vi "Begin.vi"(8 "error in":errorcluster) -> (0 "error out":errorcluster)   [LabVIEW 2018]
doc: "Called before other user functions, this VI is expected to open initial I/O refnums, load in file data, and do all program initialization. Notice that the <B>error out</B> terminal is simply used for data flow. Wiring it to other structures or subVIs ensures that this VI runs first."
uses:
  <vilib>/Rock Robotics/WPI/DriverStation/WPI_DriverStationRobotMode2.ctl
  <vilib>/Rock Robotics/WPI/Joystick/WPI_JoystickDeviceEnum.ctl
  <vilib>/Rock Robotics/WPI/Solenoid/WPI_SolenoidChannel.ctl
  <vilib>/Rock Robotics/SystemInterfaces/DIO/FPGA_DIOPWMChannel.ctl
  <vilib>/Rock Robotics/SystemInterfaces/AI/FPGA_AIChannel.ctl
  <vilib>/Rock Robotics/SystemInterfaces/spilib/spi_bus.ctl
  <vilib>/Rock Robotics/SystemInterfaces/DIO/FPGA_DIOChannel.ctl
  Robot Global Data.vi
  <vilib>/Rock Robotics/WPI/Utilities/WPI_GetSetVariantRefNum.vi
  <vilib>/Rock Robotics/WPI/Solenoid/WPI_SolenoidOpenSingle.vi
  <vilib>/Rock Robotics/WPI/MotorControl/WPI_MotorControlOpen SPARK.vi
  navx-mxp/labview/navX Library v2/IO/Open/Z900_navX_Open_SPI.vi
  Swerve/SwerveGlobals.vi
  <vilib>/Rock Robotics/WPI/Counter/WPI_CounterDigitalInputToDigitalSource.vi
  navx-mxp/labview/navX Library v2/navX Library v2.lvlib
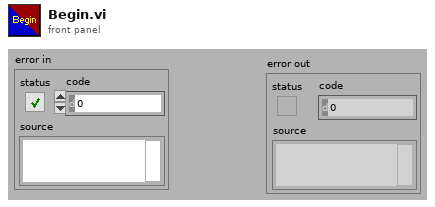
[diagram p1: front panel]
types:
  T1 = typedef "WPI_DriverStationRobotMode2.ctl" = enum16{"Autonomous Disabled", "Autonomous Enabled", "Teleop Disabled", "Teleop Enabled", "Disconnected", "Finish", "Test Disabled", "Test Enabled", "Emergency Stopped"}
  T2 = typedef "WPI_JoystickDeviceEnum.ctl" = enum16{"USB 0", "USB 1", "USB 2", "USB 3", "USB 4", "USB 5"}
  T3 = typedef "FPGA_DIOPWMChannel.ctl" = enum8{"PWM 0", "PWM 1", "PWM 2", "PWM 3", "PWM 4", "PWM 5", "PWM 6", "PWM 7", "PWM 8", "PWM 9", "PWM MXP 0", "PWM MXP 1", "PWM MXP 2", "PWM MXP 3", "PWM MXP 4", "PWM MXP 5", "PWM MXP 6", "PWM MXP 7", "PWM MXP 8", "PWM MXP 9", "Invalid"}
  T4 = typedef "WPI_SolenoidChannel.ctl" = enum8{"Solenoid 0", "Solenoid 1", "Solenoid 2", "Solenoid 3", "Solenoid 4", "Solenoid 5", "Solenoid 6", "Solenoid 7", "Invalid"}
  T5 = typedef "FPGA_AIChannel.ctl" = enum8{"AI 0", "AI 1", "AI 2", "AI 3", "AI MXP 0", "AI MXP 1", "AI MXP 2", "AI MXP 3", "Invalid"}
  T6 = typedef "spi_bus.ctl" = enum16{"SPI On-Board, CS0", "SPI On-Board, CS1", "SPI On-Board, CS2", "SPI On-Board, CS3", "SPI MXP", "Invalid"}
  T7 = typedef "WPI_JoystickDevRef.ctl" = cluster{"Device":T2}
  T8 = typedef "WPI_MotorControlDeviceRef.ctl" = cluster{"DeviceStatus":errorcluster, "Type":T9, "PWM":cluster{"PWM Channel":T3, "DeadBand":T10}, "CAN":cluster{"Device Number":u8, "SetOutput VI Ref":variant, "GetOutput VI Ref":variant, "Enable VI Ref":variant, "Disable VI Ref":variant, "Data":variant}, "Invert":bool, "DIO PWM":cluster{"PWM \"Enable\" Channel":T3, "DIOChannel":T11, "PWM Rate":dbl}}
  T9 = typedef "WPI_MotorControlType.ctl" = enum16{"PWM", "CAN", "DIO PWM"}
  T10 = typedef "WPI_PWMDeadband.ctl" = cluster{"Name":string, "maxPositivePwm":i32, "minPositivePwm":i32, "centerPwm":i32, "maxNegativePwm":i32, "minNegativePwm":i32, "angularRange":u16}
  T11 = typedef "FPGA_DIOChannel.ctl" = enum8{"DIO 0", "DIO 1", "DIO 2", "DIO 3", "DIO 4", "DIO 5", "DIO 6", "DIO 7", "DIO 8", "DIO 9", "DIO MXP 0", "DIO MXP 1", "DIO MXP 2", "DIO MXP 3", "DIO MXP 4", "DIO MXP 5", "DIO MXP 6", "DIO MXP 7", "DIO MXP 8", "DIO MXP 9", "DIO MXP 10", "DIO MXP 11", "DIO MXP 12", "DIO MXP 13", "DIO MXP 14", "DIO MXP 15", "SPI Port CS1", "SPI Port CS2", "SPI Port CS3", "SPI Port MISO", "SPI Port MOSI", "Invalid"}
  T12 = typedef "WPI_CompressorDevRef.ctl" = cluster{"DevStatus":errorcluster, "Pneumatics Control Module":u8}
  T13 = typedef "WPI_SolenoidDevRef.ctl" = cluster{"DevStatus":errorcluster, "Pneumatics Control Module":u8, "Forward Solenoid Channel":T4, "Reverse Solenoid Channel":T4}
  T14 = typedef "WPI_AnalogChannelDevRef.ctl" = cluster{"DevStatus":errorcluster, "Analog Channel":T5}
  T15 = typedef "navX Library v2.lvlib/Z900_navX_DeviceTypeDef.ctl" = cluster{"Interface":cluster{"Protocol":T16, "Update Rate (4Hz-100Hz)":u8, "navX Open TypeDef":variant}, "Notify Packet":refnum<notifier>, "Loop VI Refnum":refnum<vi>, "Ready to Close Occurrence Refnum":refnum<k4>}
  T16 = typedef "navX Library v2.lvlib/Z900_navX_ProtocolTypeDef.ctl" = enum16{"SERIAL", "I2C", "SPI"}
  T17 = cluster{"Yaw":dbl, "Roll":dbl, "Pitch":dbl, "Heading":dbl, "Fused Heading":dbl}
  T18 = typedef "WPI_DigitalInputDevRef.ctl" = cluster{"DevStatus":errorcluster, "DIO Channel":T11}
  T19 = typedef "FPGA_CounterEncoderSourceConvertionLVSourceType.ctl" = cluster{"DevStatus":errorcluster, "AnalogTriggerMode?":bool, "DigitalMode":cluster{"DIO Channel":T20}, "AnalogTriggerMode":cluster{"AnalogTriggerIndex":T21, "OutputType":T22}}
  T20 = typedef "FPGA_DIODigitalSourceChannel.ctl" = enum8{"DIO 0", "DIO 1", "DIO 2", "DIO 3", "DIO 4", "DIO 5", "DIO 6", "DIO 7", "DIO 8", "DIO 9", "DIO MXP 0", "DIO MXP 1", "DIO MXP 2", "DIO MXP 3", "DIO MXP 4", "DIO MXP 5", "DIO MXP 6", "DIO MXP 7", "DIO MXP 8", "DIO MXP 9", "DIO MXP 10", "DIO MXP 11", "DIO MXP 12", "DIO MXP 13", "DIO MXP 14", "DIO MXP 15", "SPI Port CS1", "SPI Port CS2", "SPI Port CS3", "SPI Port MISO", "SPI Port MOSI", "Disabled"}
  T21 = typedef "FPGA_AnalogTriggerIndex.ctl" = enum8{"Trig 0", "Trig 1", "Trig 2", "Trig 3", "Trig 4", "Trig 5", "Trig 6", "Trig 7", "Invalid"}
  T22 = typedef "FPGA_AnalogTriggerOutType.ctl" = enum16{"InWindow", "TriggerState", "Rising", "Falling"}
  T23 = typedef "WPI_EncoderDevRef.ctl" = cluster{"DevStatus":errorcluster, "EncoderIndex":T24, "CounterIndex":T25, "DistancePerCount":dbl, "Decoding Type":T26}
  T24 = typedef "FPGA_EncoderIdx.ctl" = enum8{"Enc 0", "Enc 1", "Enc 2", "Enc 3", "Enc 4", "Enc 5", "Enc 6", "Enc 7", "Invalid"}
  T25 = typedef "FPGA_CounterCtrSystemIndex.ctl" = enum8{"Ctr 0", "Ctr 1", "Ctr 2", "Ctr 3", "Ctr 4", "Ctr 5", "Ctr 6", "Ctr 7", "Invalid"}
  T26 = typedef "WPI_EncoderType.ctl" = enum16{"1x", "2x", "4x"}
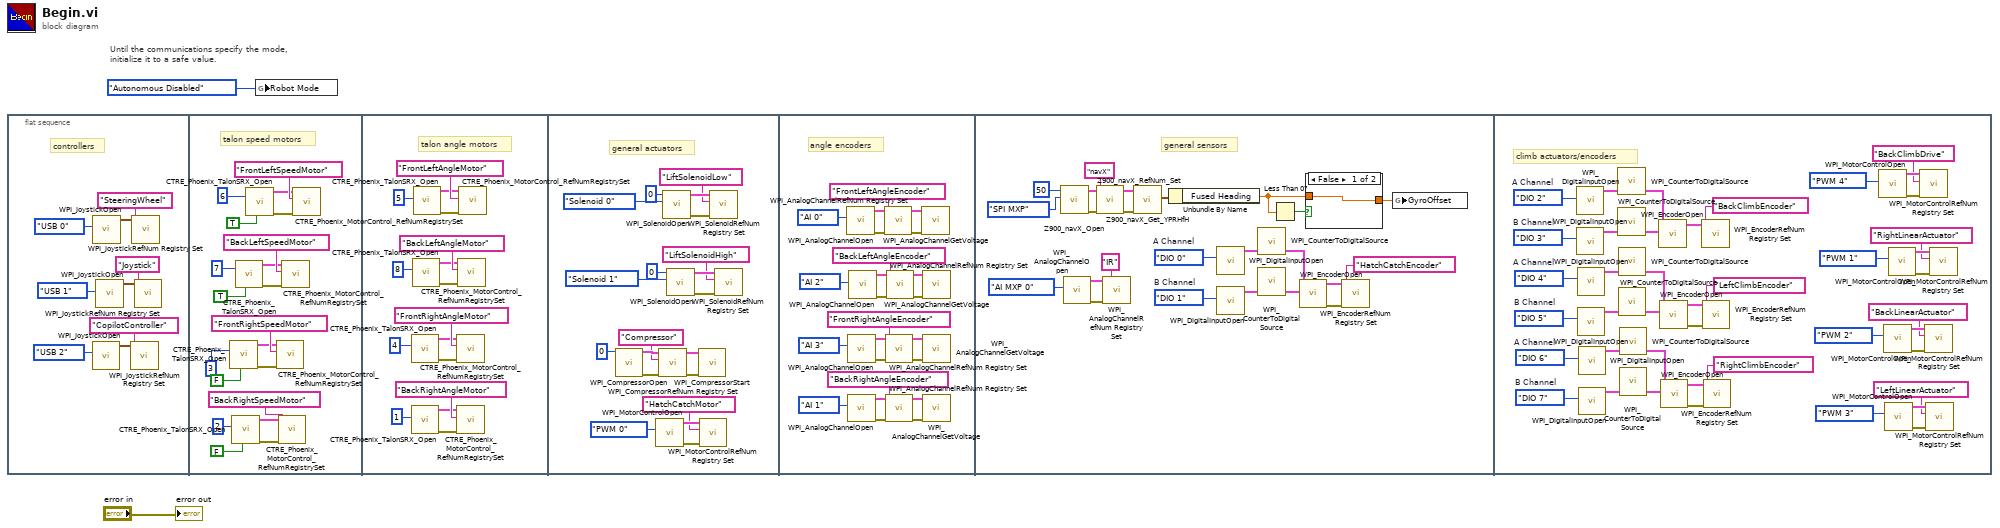
[diagram p0: block diagram]
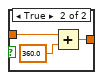
[diagram p2: hidden frame]
diagram:
  # "Until the communications specify the mode,\ninitialize it to a safe value."
  n1 = flat-sequence {
    frame #0 {
      # "controllers"
      n2 = call <vilib>:"WPI_JoystickOpen.vi"("JoystickDevice"=WPI_JoystickDeviceEnum."USB 2") -> ("JoystickDevRef"=w5:T7)  [unwired: 10 in]
      n3 = call <vilib>:"WPI_JoystickOpen.vi"("JoystickDevice"=WPI_JoystickDeviceEnum."USB 0") -> ("JoystickDevRef"=w11:T7)  [unwired: 10 in]
      n4 = call <vilib>:"WPI_JoystickOpen.vi"("JoystickDevice"=WPI_JoystickDeviceEnum."USB 1") -> ("JoystickDevRef"=w8:T7)  [unwired: 10 in]
      n5 = call <vilib>:"WPI_JoystickRefNum Registry Set.vi"("refnum name"="CopilotController", "JoystickDevRef"=w5) -> ()  [unwired: 8 in, 2 out]
      n6 = call <vilib>:"WPI_JoystickRefNum Registry Set.vi"("refnum name"="SteeringWheel", "JoystickDevRef"=w11) -> ()  [unwired: 8 in, 2 out]
      n7 = call <vilib>:"WPI_JoystickRefNum Registry Set.vi"("refnum name"="Joystick", "JoystickDevRef"=w8) -> ()  [unwired: 8 in, 2 out]
    }
    frame #1 {
      # "talon speed motors"
      n8 = call <vilib>:"CTRE_Phoenix_TalonSRX_Open.vi"("Invert"=FALSE, "Device Number"=u8 3) -> ("error out"=w20:errorcluster, "CAN Talon SRX Ref"=w21:T8)  [unwired: 8 in]
      n9 = call <vilib>:"CTRE_Phoenix_TalonSRX_Open.vi"("Invert"=FALSE, "Device Number"=u8 2) -> ("error out"=w22:errorcluster, "CAN Talon SRX Ref"=w23:T8)  [unwired: 8 in]
      n10 = call <vilib>:"CTRE_Phoenix_TalonSRX_Open.vi"("Invert"=TRUE, "Device Number"=u8 7) -> ("error out"=w18:errorcluster, "CAN Talon SRX Ref"=w19:T8)  [unwired: 8 in]
      n11 = call <vilib>:"CTRE_Phoenix_TalonSRX_Open.vi"("Invert"=TRUE, "Device Number"=u8 6) -> ("error out"=w16:errorcluster, "CAN Talon SRX Ref"=w17:T8)  [unwired: 8 in]
      n12 = call <vilib>:"CTRE_Phoenix_MotorControl_RefNumRegistrySet.vi"("error in (no error)"=w20, "refnum name"="FrontRightSpeedMotor", "PhoenixMotorControlDevRef"=w21) -> ()  [unwired: 7 in, 2 out]
      n13 = call <vilib>:"CTRE_Phoenix_MotorControl_RefNumRegistrySet.vi"("error in (no error)"=w22, "refnum name"="BackRightSpeedMotor", "PhoenixMotorControlDevRef"=w23) -> ()  [unwired: 7 in, 2 out]
      n14 = call <vilib>:"CTRE_Phoenix_MotorControl_RefNumRegistrySet.vi"("error in (no error)"=w18, "refnum name"="BackLeftSpeedMotor", "PhoenixMotorControlDevRef"=w19) -> ()  [unwired: 7 in, 2 out]
      n15 = call <vilib>:"CTRE_Phoenix_MotorControl_RefNumRegistrySet.vi"("error in (no error)"=w16, "refnum name"="FrontLeftSpeedMotor", "PhoenixMotorControlDevRef"=w17) -> ()  [unwired: 7 in, 2 out]
    }
    frame #2 {
      # "talon angle motors"
      n16 = call <vilib>:"CTRE_Phoenix_TalonSRX_Open.vi"("Device Number"=u8 4) -> ("error out"=w34:errorcluster, "CAN Talon SRX Ref"=w35:T8)  [unwired: 9 in]
      n17 = call <vilib>:"CTRE_Phoenix_TalonSRX_Open.vi"("Device Number"=u8 1) -> ("error out"=w32:errorcluster, "CAN Talon SRX Ref"=w33:T8)  [unwired: 9 in]
      n18 = call <vilib>:"CTRE_Phoenix_TalonSRX_Open.vi"("Device Number"=u8 8) -> ("error out"=w36:errorcluster, "CAN Talon SRX Ref"=w37:T8)  [unwired: 9 in]
      n19 = call <vilib>:"CTRE_Phoenix_TalonSRX_Open.vi"("Device Number"=u8 5) -> ("error out"=w38:errorcluster, "CAN Talon SRX Ref"=w39:T8)  [unwired: 9 in]
      n20 = call <vilib>:"CTRE_Phoenix_MotorControl_RefNumRegistrySet.vi"("error in (no error)"=w34, "refnum name"="FrontRightAngleMotor", "PhoenixMotorControlDevRef"=w35) -> ()  [unwired: 7 in, 2 out]
      n21 = call <vilib>:"CTRE_Phoenix_MotorControl_RefNumRegistrySet.vi"("error in (no error)"=w32, "refnum name"="BackRightAngleMotor", "PhoenixMotorControlDevRef"=w33) -> ()  [unwired: 7 in, 2 out]
      n22 = call <vilib>:"CTRE_Phoenix_MotorControl_RefNumRegistrySet.vi"("error in (no error)"=w36, "refnum name"="BackLeftAngleMotor", "PhoenixMotorControlDevRef"=w37) -> ()  [unwired: 7 in, 2 out]
      n23 = call <vilib>:"CTRE_Phoenix_MotorControl_RefNumRegistrySet.vi"("error in (no error)"=w38, "refnum name"="FrontLeftAngleMotor", "PhoenixMotorControlDevRef"=w39) -> ()  [unwired: 7 in, 2 out]
    }
    frame #3 {
      # "general actuators"
      n24 = call <vilib>:"WPI_CompressorOpen.vi"("Pneumatics Control Module (0)"=u8 0) -> ("CompressorDevRef"=w67:T12, "error out"=w52:errorcluster)  [unwired: 13 in]
      n25 = call-poly <vilib>:"WPI_MotorControlOpen.vi"("PWM Channel"=FPGA_DIOPWMChannel."PWM 0") -> ("error out"=w56:errorcluster, "MotorControlDeviceRef"=w55:T8)  [unwired: 9 in]
      n26 = call <vilib>:"WPI_CompressorRefNum Registry Set.vi"("error in (no error)"=w52, "refnum name"="Compressor", "CompressorDevRef"=w67) -> ("error out"=w48:errorcluster, "CompressorDevRef"=w49:T12)  [unwired: 7 in]
      n27 = call-poly <vilib>:"WPI_SolenoidOpen.vi"("Solenoid Channel"=WPI_SolenoidChannel."Solenoid 0", "Pneumatics Control Module (0)"=u8 0) -> ("error out"=w50:errorcluster, "SolenoidDevRef"=w66:T13)  [unwired: 8 in]
      n28 = call-poly <vilib>:"WPI_SolenoidOpen.vi"("Solenoid Channel"=WPI_SolenoidChannel."Solenoid 1", "Pneumatics Control Module (0)"=u8 0) -> ("error out"=w51:errorcluster, "SolenoidDevRef"=w63:T13)  [unwired: 8 in]
      n29 = call <vilib>:"WPI_CompressorStart.vi"("error in (no error)"=w48, "CompressorDevRef"=w49) -> ()  [unwired: 8 in, 2 out]
      n30 = call <vilib>:"WPI_MotorControlRefNum Registry Set.vi"("error in (no error)"=w56, "refnum name"="HatchCatchMotor", "MotorControlDevRef"=w55) -> ()  [unwired: 7 in, 2 out]
      n31 = call <vilib>:"WPI_SolenoidRefNum Registry Set.vi"("error in (no error)"=w50, "refnum name"="LiftSolenoidLow", "SolenoidDevRef"=w66) -> ()  [unwired: 7 in, 2 out]
      n32 = call <vilib>:"WPI_SolenoidRefNum Registry Set.vi"("error in (no error)"=w51, "refnum name"="LiftSolenoidHigh", "SolenoidDevRef"=w63) -> ()  [unwired: 7 in, 2 out]
    }
    frame #4 {
      # "angle encoders"
      n33 = call <vilib>:"WPI_AnalogChannelOpen.vi"("Analog Channel"=FPGA_AIChannel."AI 0") -> ("error out"=w90:errorcluster, "AIDeviceRef"=w91:T14)  [unwired: 9 in]
      n34 = call <vilib>:"WPI_AnalogChannelOpen.vi"("Analog Channel"=FPGA_AIChannel."AI 3") -> ("error out"=w82:errorcluster, "AIDeviceRef"=w83:T14)  [unwired: 9 in]
      n35 = call <vilib>:"WPI_AnalogChannelOpen.vi"("Analog Channel"=FPGA_AIChannel."AI 1") -> ("error out"=w78:errorcluster, "AIDeviceRef"=w79:T14)  [unwired: 9 in]
      n36 = call <vilib>:"WPI_AnalogChannelOpen.vi"("Analog Channel"=FPGA_AIChannel."AI 2") -> ("error out"=w86:errorcluster, "AIDeviceRef"=w87:T14)  [unwired: 9 in]
      n37 = call <vilib>:"WPI_AnalogChannelRefNum Registry Set.vi"("error in (no error)"=w90, "refnum name"="FrontLeftAngleEncoder", "AIDeviceRef"=w91) -> ("error out"=w74:errorcluster, "AIDeviceRef"=w75:T14)  [unwired: 7 in]
      n38 = call <vilib>:"WPI_AnalogChannelRefNum Registry Set.vi"("error in (no error)"=w82, "refnum name"="FrontRightAngleEncoder", "AIDeviceRef"=w83) -> ("error out"=w70:errorcluster, "AIDeviceRef"=w71:T14)  [unwired: 7 in]
      n39 = call <vilib>:"WPI_AnalogChannelRefNum Registry Set.vi"("error in (no error)"=w78, "refnum name"="BackRightAngleEncoder", "AIDeviceRef"=w79) -> ("error out"=w68:errorcluster, "AIDeviceRef"=w69:T14)  [unwired: 7 in]
      n40 = call <vilib>:"WPI_AnalogChannelRefNum Registry Set.vi"("error in (no error)"=w86, "refnum name"="BackLeftAngleEncoder", "AIDeviceRef"=w87) -> ("error out"=w72:errorcluster, "AIDeviceRef"=w73:T14)  [unwired: 7 in]
      n41 = call <vilib>:"WPI_AnalogChannelGetVoltage.vi"("error in (no error)"=w74, "AIDeviceRef"=w75) -> ()  [unwired: 7 in, 3 out]
      n42 = call <vilib>:"WPI_AnalogChannelGetVoltage.vi"("error in (no error)"=w72, "AIDeviceRef"=w73) -> ()  [unwired: 7 in, 3 out]
      n43 = call <vilib>:"WPI_AnalogChannelGetVoltage.vi"("error in (no error)"=w70, "AIDeviceRef"=w71) -> ()  [unwired: 7 in, 3 out]
      n44 = call <vilib>:"WPI_AnalogChannelGetVoltage.vi"("error in (no error)"=w68, "AIDeviceRef"=w69) -> ()  [unwired: 7 in, 3 out]
    }
    frame #5 {
      w100 = FPGA_DIOChannel."DIO 1"  # B Channel
      w99 = FPGA_DIOChannel."DIO 0"  # A Channel
      # "general sensors"
      n45 = call-poly "Z900_navX_Open.vi"("SPI Bus"=spi_bus."SPI MXP", "Update Rate (4Hz-60Hz)"=u8 50) -> ("error out"=w115:errorcluster, "navX Device"=w114:T15)  [unwired: 8 in]
      n46 = call <vilib>:"WPI_AnalogChannelOpen.vi"("Analog Channel"=FPGA_AIChannel."AI MXP 0") -> ("error out"=w103:errorcluster, "AIDeviceRef"=w104:T14)  [unwired: 9 in]
      n47 = call "Z900_navX_RefNum_Set.vi"("error in (no error)"=w115, "refnum name"="navX", "navX Device"=w114) -> ("error out"=w109:errorcluster, "navX Device"=w110:T15)  [unwired: 7 in]
      n48 = call <vilib>:"WPI_AnalogChannelRefNum Registry Set.vi"("error in (no error)"=w103, "refnum name"="IR", "AIDeviceRef"=w104) -> ()  [unwired: 7 in, 2 out]
      n49 = call "Z900_navX_Get_YPRHfH.vi"("error in (no error)"=w109, "navX Device"=w110) -> ("YRPHfH"=w111:T17)  [unwired: 6 in, 3 out]
      n50 = Unbundle By Name(w111) -> ("Fused Heading"=w107:dbl)
      n51 = call <vilib>:"WPI_DigitalInputOpen.vi"("DIO Channel"=w99) -> ("DigitalInputDevRef"=w96:T18)  [unwired: 1 in, 9 out]
      n52 = call <vilib>:"WPI_DigitalInputOpen.vi"("DIO Channel"=w100) -> ("DigitalInputDevRef"=w97:T18)  [unwired: 1 in, 9 out]
      n53 = call-poly <vilib>:"WPI_CounterToDigitalSource.vi"("DigitalInputDevRef"=w96) -> ("Digital Source"=w95:T19)  [unwired: 6 out]
      n54 = call-poly <vilib>:"WPI_CounterToDigitalSource.vi"("DigitalInputDevRef"=w97) -> ("Digital Source"=w98:T19)  [unwired: 6 out]
      n55 = Less Than 0?(x=w107) -> (x < 0?=w108:bool)
      n56 = call <vilib>:"WPI_EncoderOpen.vi"("BSource"=w98, "ASource"=w95) -> ("error out"=w94:errorcluster, "EncoderDevRef"=w93:T23)  [unwired: 6 in, 2 out]
      n57 = case shown="False" w108 {
        tunnel: w107 -> [w116 w119]
        tunnel: [w116 w117] -> w106
        frame False {
        }
        frame True {
          n58 = Add(x=w119, y=360.0) -> (x+y=w117:dbl)
        }
      }
      n59 = call <vilib>:"WPI_EncoderRefNum Registry Set.vi"("error in (no error)"=w94, "refnum name"="HatchCatchEncoder", "EncoderDevRef"=w93) -> ()  [unwired: 7 in, 2 out]
      n60 = global write "SwerveGlobals.vi" "GyroOffset"(w106) -> ()
    }
    frame #6 {
      w137 = FPGA_DIOChannel."DIO 7"  # B Channel
      w136 = FPGA_DIOChannel."DIO 6"  # A Channel
      w146 = FPGA_DIOChannel."DIO 5"  # B Channel
      w145 = FPGA_DIOChannel."DIO 4"  # A Channel
      w155 = FPGA_DIOChannel."DIO 3"  # B Channel
      w154 = FPGA_DIOChannel."DIO 2"  # A Channel
      # "climb actuators/encoders"
      n61 = call <vilib>:"WPI_DigitalInputOpen.vi"("DIO Channel"=w154) -> ("DigitalInputDevRef"=w159:T18)  [unwired: 1 in, 9 out]
      n62 = call <vilib>:"WPI_DigitalInputOpen.vi"("DIO Channel"=w155) -> ("DigitalInputDevRef"=w160:T18)  [unwired: 1 in, 9 out]
      n63 = call <vilib>:"WPI_DigitalInputOpen.vi"("DIO Channel"=w145) -> ("DigitalInputDevRef"=w150:T18)  [unwired: 1 in, 9 out]
      n64 = call <vilib>:"WPI_DigitalInputOpen.vi"("DIO Channel"=w146) -> ("DigitalInputDevRef"=w149:T18)  [unwired: 1 in, 9 out]
      n65 = call <vilib>:"WPI_DigitalInputOpen.vi"("DIO Channel"=w136) -> ("DigitalInputDevRef"=w141:T18)  [unwired: 1 in, 9 out]
      n66 = call <vilib>:"WPI_DigitalInputOpen.vi"("DIO Channel"=w137) -> ("DigitalInputDevRef"=w140:T18)  [unwired: 1 in, 9 out]
      n67 = call-poly <vilib>:"WPI_CounterToDigitalSource.vi"("DigitalInputDevRef"=w159) -> ("Digital Source"=w158:T19)  [unwired: 6 out]
      n68 = call-poly <vilib>:"WPI_CounterToDigitalSource.vi"("DigitalInputDevRef"=w160) -> ("Digital Source"=w161:T19)  [unwired: 6 out]
      n69 = call-poly <vilib>:"WPI_CounterToDigitalSource.vi"("DigitalInputDevRef"=w150) -> ("Digital Source"=w151:T19)  [unwired: 6 out]
      n70 = call-poly <vilib>:"WPI_CounterToDigitalSource.vi"("DigitalInputDevRef"=w149) -> ("Digital Source"=w148:T19)  [unwired: 6 out]
      n71 = call-poly <vilib>:"WPI_CounterToDigitalSource.vi"("DigitalInputDevRef"=w141) -> ("Digital Source"=w142:T19)  [unwired: 6 out]
      n72 = call-poly <vilib>:"WPI_CounterToDigitalSource.vi"("DigitalInputDevRef"=w140) -> ("Digital Source"=w139:T19)  [unwired: 6 out]
      n73 = call <vilib>:"WPI_EncoderOpen.vi"("BSource"=w161, "ASource"=w158) -> ("EncoderDevRef"=w157:T23)  [unwired: 6 in, 3 out]
      n74 = call <vilib>:"WPI_EncoderOpen.vi"("BSource"=w148, "ASource"=w151) -> ("error out"=w152:errorcluster, "EncoderDevRef"=w153:T23)  [unwired: 6 in, 2 out]
      n75 = call <vilib>:"WPI_EncoderOpen.vi"("BSource"=w139, "ASource"=w142) -> ("error out"=w143:errorcluster, "EncoderDevRef"=w144:T23)  [unwired: 6 in, 2 out]
      n76 = call <vilib>:"WPI_EncoderRefNum Registry Set.vi"("refnum name"="BackClimbEncoder", "EncoderDevRef"=w157) -> ()  [unwired: 8 in, 2 out]
      n77 = call <vilib>:"WPI_EncoderRefNum Registry Set.vi"("error in (no error)"=w152, "refnum name"="LeftClimbEncoder", "EncoderDevRef"=w153) -> ()  [unwired: 7 in, 2 out]
      n78 = call <vilib>:"WPI_EncoderRefNum Registry Set.vi"("error in (no error)"=w143, "refnum name"="RightClimbEncoder", "EncoderDevRef"=w144) -> ()  [unwired: 7 in, 2 out]
      n79 = call-poly <vilib>:"WPI_MotorControlOpen.vi"("PWM Channel"=FPGA_DIOPWMChannel."PWM 4") -> ("error out"=w129:errorcluster, "MotorControlDeviceRef"=w128:T8)  [unwired: 9 in]
      n80 = call-poly <vilib>:"WPI_MotorControlOpen.vi"("PWM Channel"=FPGA_DIOPWMChannel."PWM 2") -> ("error out"=w131:errorcluster, "MotorControlDeviceRef"=w130:T8)  [unwired: 9 in]
      n81 = call-poly <vilib>:"WPI_MotorControlOpen.vi"("PWM Channel"=FPGA_DIOPWMChannel."PWM 3") -> ("error out"=w133:errorcluster, "MotorControlDeviceRef"=w132:T8)  [unwired: 9 in]
      n82 = call-poly <vilib>:"WPI_MotorControlOpen.vi"("PWM Channel"=FPGA_DIOPWMChannel."PWM 1") -> ("error out"=w135:errorcluster, "MotorControlDeviceRef"=w134:T8)  [unwired: 9 in]
      n83 = call <vilib>:"WPI_MotorControlRefNum Registry Set.vi"("error in (no error)"=w129, "refnum name"="BackClimbDrive", "MotorControlDevRef"=w128) -> ()  [unwired: 7 in, 2 out]
      n84 = call <vilib>:"WPI_MotorControlRefNum Registry Set.vi"("error in (no error)"=w131, "refnum name"="BackLinearActuator", "MotorControlDevRef"=w130) -> ()  [unwired: 7 in, 2 out]
      n85 = call <vilib>:"WPI_MotorControlRefNum Registry Set.vi"("error in (no error)"=w133, "refnum name"="LeftLinearActuator", "MotorControlDevRef"=w132) -> ()  [unwired: 7 in, 2 out]
      n86 = call <vilib>:"WPI_MotorControlRefNum Registry Set.vi"("error in (no error)"=w135, "refnum name"="RightLinearActuator", "MotorControlDevRef"=w134) -> ()  [unwired: 7 in, 2 out]
    }
  }
  n87 = global write "Robot Global Data.vi" "Robot Mode"(WPI_DriverStationRobotMode2."Autonomous Disabled" ("Robot Mode")) -> ()
  "error out" <- "error in"
